vi "S2C_FPGA_InterfaceGlobals.vi"() -> ()   [LabVIEW 2015]
panel:
  in  "C0/AI7":dbl min=-10.0 max=10.0 step=0.00048828125 format="%#.6g"
  in  "C0/AO7":dbl min=-10.0 max=10.0
  in  "C0/AI6":dbl min=-10.0 max=10.0 step=0.00048828125 format="%#.6g"
  in  "C0/AI5":dbl min=-10.0 max=10.0 step=0.00048828125 format="%#.6g"
  in  "C0/AI4":dbl min=-10.0 max=10.0 step=0.00048828125 format="%#.6g"
  in  "C0/AI3":dbl min=-10.0 max=10.0 step=0.00048828125 format="%#.6g"
  in  "C0/AI2":dbl min=-10.0 max=10.0 step=0.00048828125 format="%#.6g"
  in  "C0/AI1":dbl min=-10.0 max=10.0 step=0.00048828125 format="%#.6g"
  in  "C0/AI0":dbl min=-10.0 max=10.0 format="%#.6f"
  in  "C0/AO6":dbl min=-10.0 max=10.0
  in  "C0/AO5":dbl min=-10.0 max=10.0
  in  "C0/AO4":dbl min=-10.0 max=10.0
  in  "C0/AO3":dbl min=-10.0 max=10.0
  in  "C0/AO2":dbl min=-10.0 max=10.0
  in  "C0/AO1":dbl min=-10.0 max=10.0
  in  "C0/AO0":dbl min=-10.0 max=10.0
  out "C0_P1 Out":u8 format="%08b"
  out "C0_P0 Out":u8 format="%08b"
  out "C2_P4 Out":u8 format="%08b"
  out "C2_P3 Out":u8 format="%08b"
  out "C2_P2 Out":u8 format="%08b"
  out "C2_P1 Out":u8 format="%08b"
  out "C2_P0 Out":u8 format="%08b"
  out "C1_P4 Out":u8 format="%08b"
  out "C1_P3 Out":u8 format="%08b"
  out "C1_P2 Out":u8 format="%08b"
  out "C1_P1 Out":u8 format="%08b"
  out "C1_P0 Out":u8 format="%08b"
  out "C2/P4/B7":bool
  out "C2/P4/B6":bool
  out "C2/P4/B5":bool
  out "C2/P4/B4":bool
  out "C2/P4/B3":bool
  out "C2/P4/B2":bool
  out "C2/P4/B1":bool
  out "C2/P4/B0":bool
  out "C2/P3/B7":bool
  out "C2/P3/B6":bool
  out "C2/P3/B5":bool
  out "C2/P3/B4":bool
  out "C2/P3/B3":bool
  out "C2/P3/B2":bool
  out "C2/P3/B1":bool
  out "C2/P3/B0":bool
  out "C2/P2/B7":bool
  out "C2/P2/B6":bool
  out "C2/P2/B5":bool
  out "C2/P2/B4":bool
  out "C2/P2/B3":bool
  out "C2/P2/B2":bool
  out "C2/P2/B1":bool
  out "C2/P2/B0":bool
  out "C2/P1/B7":bool
  out "C2/P1/B6":bool
  out "C2/P1/B5":bool
  out "C2/P1/B4":bool
  out "C2/P1/B3":bool
  out "C2/P1/B2":bool
  out "C2/P1/B1":bool
  out "C2/P1/B0":bool
  out "C2/P0/B7":bool
  out "C2/P0/B6":bool
  out "C2/P0/B5":bool
  out "C2/P0/B4":bool
  out "C2/P0/B3":bool
  out "C2/P0/B2":bool
  out "C2/P0/B1":bool
  out "C2/P0/B0":bool
  out "C1/P4/B7":bool
  out "C1/P4/B6":bool
  out "C1/P4/B5":bool
  out "C1/P4/B4":bool
  out "C1/P4/B3":bool
  out "C1/P4/B2":bool
  out "C1/P4/B1":bool
  out "C1/P4/B0":bool
  out "C1/P3/B7":bool
  out "C1/P3/B6":bool
  out "C1/P3/B5":bool
  out "C1/P3/B4":bool
  out "C1/P3/B3":bool
  out "C1/P3/B2":bool
  out "C1/P3/B1":bool
  out "C1/P3/B0":bool
  out "C1/P2/B7":bool
  out "C1/P2/B6":bool
  out "C1/P2/B5":bool
  out "C1/P2/B4":bool
  out "C1/P2/B3":bool
  out "C1/P2/B2":bool
  out "C1/P2/B1":bool
  out "C1/P2/B0":bool
  out "C1/P1/B7":bool
  out "C1/P1/B6":bool
  out "C1/P1/B5":bool
  out "C1/P1/B4":bool
  out "C1/P1/B3":bool
  out "C1/P1/B2":bool
  out "C1/P1/B1":bool
  out "C1/P1/B0":bool
  out "C1/P0/B7":bool
  out "C1/P0/B6":bool
  out "C1/P0/B5":bool
  out "C1/P0/B4":bool
  out "C1/P0/B3":bool
  out "C1/P0/B2":bool
  out "C1/P0/B1":bool
  out "C1/P0/B0":bool
  out "C0/P1/B7":bool
  out "C0/P1/B6":bool
  out "C0/P1/B5":bool
  out "C0/P1/B4":bool
  out "C0/P1/B3":bool
  out "C0/P1/B2":bool
  out "C0/P1/B1":bool
  out "C0/P1/B0":bool
  out "C0/P0/B7":bool
  out "C0/P0/B6":bool
  out "C0/P0/B5":bool
  out "C0/P0/B4":bool
  out "C0/P0/B3":bool
  out "C0/P0/B2":bool
  out "C0/P0/B1":bool
  out "C0/P0/B0":bool
  in  "Restrictions":string[][](array[string])
  out "Restrict?":bool
  in  "FPGA_Ref":refnum<k20>
  out "DisableUnused?":bool
  in  "Settings File":path
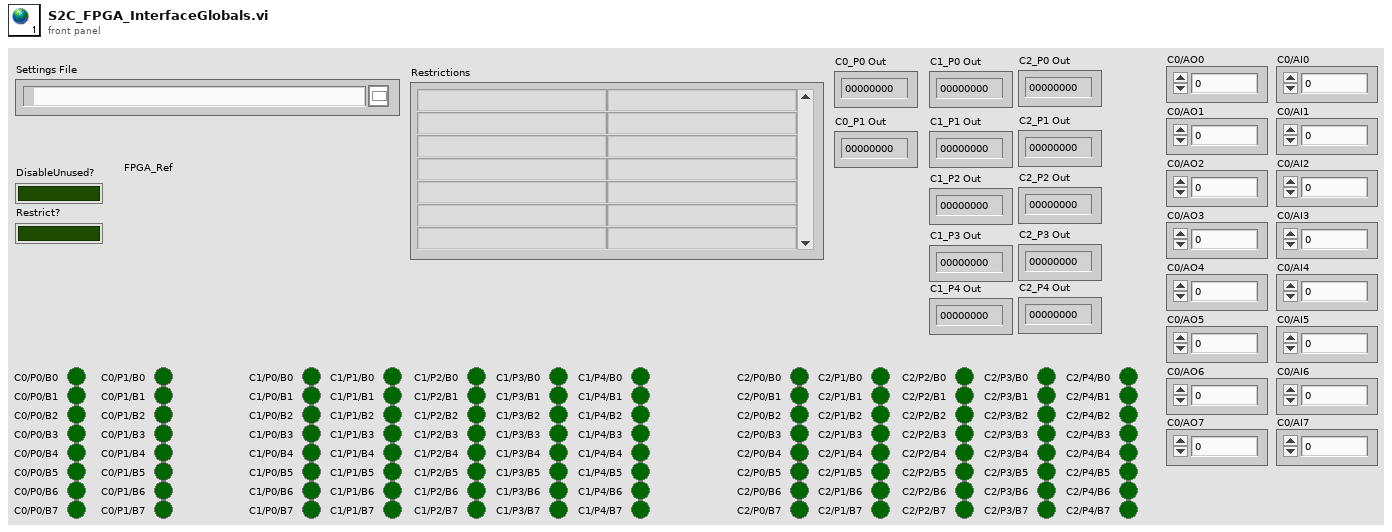
[diagram p1: front panel]
diagram:
